vi "PH_SHS_Analysis.Draw Image.vi"(0 "i ref in":refnum<vi>, 2 "Cam Image":T1, 5 "error in (no error)":errorcluster) -> (14 "i ref out":refnum<vi>, 19 "error out":errorcluster)   [LabVIEW 2014, in "PH_SHS_Analysis.lvlib"]
doc: "This VI draws the image to the GUI. Depending on the sequencer state, it writes the images also to the attributes or calculates the pixel sum."
uses:
  PH_SHS_Analysis.lvlib
  <vilib>/vision/Image Controls.llb/IMAQ Image.ctl
  <vilib>/vision/NI_Vision_Development_Module.lvlib
  User/Eisenbarth/SHS_v4/SHS_Analysis/SHS_Analysis.lvlib
  User/Eisenbarth/SHS_v4/SHS_Common/SHS_Common.lvlib
  PH_Img_BaseClass/PH_Img_BaseClass.lvlib
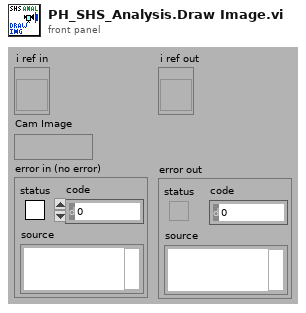
[diagram p1: front panel]
types:
  T1 = typedef "IMAQ Image.ctl" = refnum<image>
  T2 = typedef "Image Type" = u32
  T3 = typedef "PH_Img_BaseClass.lvlib/PH_Img_BaseClass.i attribute.ctl" = cluster{"GUI Refs":T4, "Timeout Image [ms]":i32, "Default Periodic Period [ms]":i32, "Camera":cluster{"Instancename":string, "Notifier":refnum<notifier>}, "Palette":T5, "Cam Settings":cluster{"Cam ID":string, "Gain":dbl, "Brightness":dbl, "Shutter":dbl, "Cam Info Failure":bool, "Mode":i32}}
  T4 = typedef "PH_Img_BaseClass.lvlib/PH_Img_BaseClass.GUI Refs.ctl" = cluster{"Timeout":refnum<vi>, "Image":refnum<vi>, "Palette":refnum<vi>, "Timeout Set":refnum<vi>}
  T5 = typedef "PH_Img_BaseClass.lvlib/PH_Img_BaseClass.Palette.ctl" = i32
  T6 = typedef "PH_SHS_Analysis.lvlib/PH_SHS_Analysis.i attribute.ctl" = cluster{"GUI Refs":cluster{"Delete":refnum<vi>, "Global On":refnum<vi>, "Cam Source":refnum<vi>, "Calibration Data File":refnum<vi>, "Calibration status":refnum<vi>, "Show overlay":refnum<vi>, "SHS Device Config":refnum<vi>, "Result":refnum<vi>, "Consider Tilt":refnum<vi>, "Working Reference":refnum<vi>, "Remove Tilt":refnum<vi>, "Take Cali  Reference":refnum<vi>, "Publishing Data Status":refnum<vi>, "Calibration Data":refnum<vi>}, "Calibration":cluster{"Status":T7, "Data":T8, "File":path}, "Result":T13, "Image":T1, "SHS Device Config":T16, "Show Overlay":bool, "GradientZernikeMatrix":dbl[][], "Consider Tilt":bool, "Working Reference":T9, "Zernicke Service ID":i32, "PSDB Image":T1}
  T7 = typedef "PH_StatusHandler.lvlib/PH_StatusHandler.Status.ctl" = i16
  T8 = typedef "PH_SHS_Analysis_Calibrator.lvlib/PH_SHS_Analysis_Calibrator.Analysis Calibration Data.ctl" = cluster{"Date":string, "Time":string, "Cam Settings":cluster{"Cam ID":string, "Gain":dbl, "Brightness":dbl, "Shutter":dbl, "Cam Error":bool, "Mode":i32}, "SHS Reference Result":T9, "Pixel Size":dbl, "MLA Pitch":dbl, "Method":enum16{"automatic", "manual"}, "Calibration Data calculated":bool, "No Problems at calculation?":bool, "error out":errorcluster}
  T9 = typedef "SHS_Common.lvlib/SHSReference.ctl" = cluster{"Reference":T10[][], "Lens Array Pitch [px]":dbl}
  T10 = typedef "SHS_Common.lvlib/ReferencePoint.ctl" = cluster{"Rect":T11, "Point":T12}
  T11 = typedef "SHS_Common.lvlib/Rectangle.ctl" = cluster{"Left":i32, "Top":i32, "Right":i32, "Bottom":i32}
  T12 = typedef "SHS_Common.lvlib/Point.ctl" = cluster{"x":dbl, "y":dbl, "valid?":bool, "weight":dbl}
  T13 = typedef "PH_SHS_Analysis.lvlib/PH_SHS_Analysis.Result.ctl" = cluster{"Time Stamp":timestamp, "Zernike Coefficients":T14, "PtV [lambda]":dbl, "Shifts":T15, "Measurement Quality":cluster{dbl, dbl, dbl}, "Measurement valid?":bool}
  T14 = typedef "PH_SHS_Analysis.lvlib/PH_SHS_Analysis.Zernike Coefficients.ctl" = cluster{"Tilt x":dbl, "Tilt y":dbl, "Defocus":dbl, "Astig 0°":dbl, "Astig 45°":dbl, "Coma x":dbl, "Coma y":dbl, "Spherical":dbl, "Trefoil 0°":dbl, "Trefoil 30°":dbl, "2nd Astig 0°":dbl, "2nd Astig 45°":dbl, "2nd Coma x":dbl, "2nd Coma y":dbl, "2nd Spherical":dbl}
  T15 = typedef "SHS_Common.lvlib/Shifts.ctl" = T12[][]
  T16 = typedef "SHS_Analysis.lvlib/SHS_DeviceConfig.ctl" = cluster{"focal length [m]":dbl, "pixel size [m/px]":dbl, "wavelength [m]":dbl}
  T17 = enum8{"Enabled", "Disabled", "Disabled and Grayed Out"}
  T18 = cluster{"Zernike Coeffcients[0]":dbl, "Zernike Coeffcients[1]":dbl, "Zernike Coeffcients[2]":dbl, "Zernike Coeffcients[3]":dbl, "Zernike Coeffcients[4]":dbl, "Zernike Coeffcients[5]":dbl, "Zernike Coeffcients[6]":dbl, "Zernike Coeffcients[7]":dbl, "Zernike Coeffcients[8]":dbl, "Zernike Coeffcients[9]":dbl, "Zernike Coeffcients[10]":dbl, "Zernike Coeffcients[11]":dbl, "Zernike Coeffcients[12]":dbl, "Zernike Coeffcients[13]":dbl, "Zernike Coeffcients[14]":dbl}
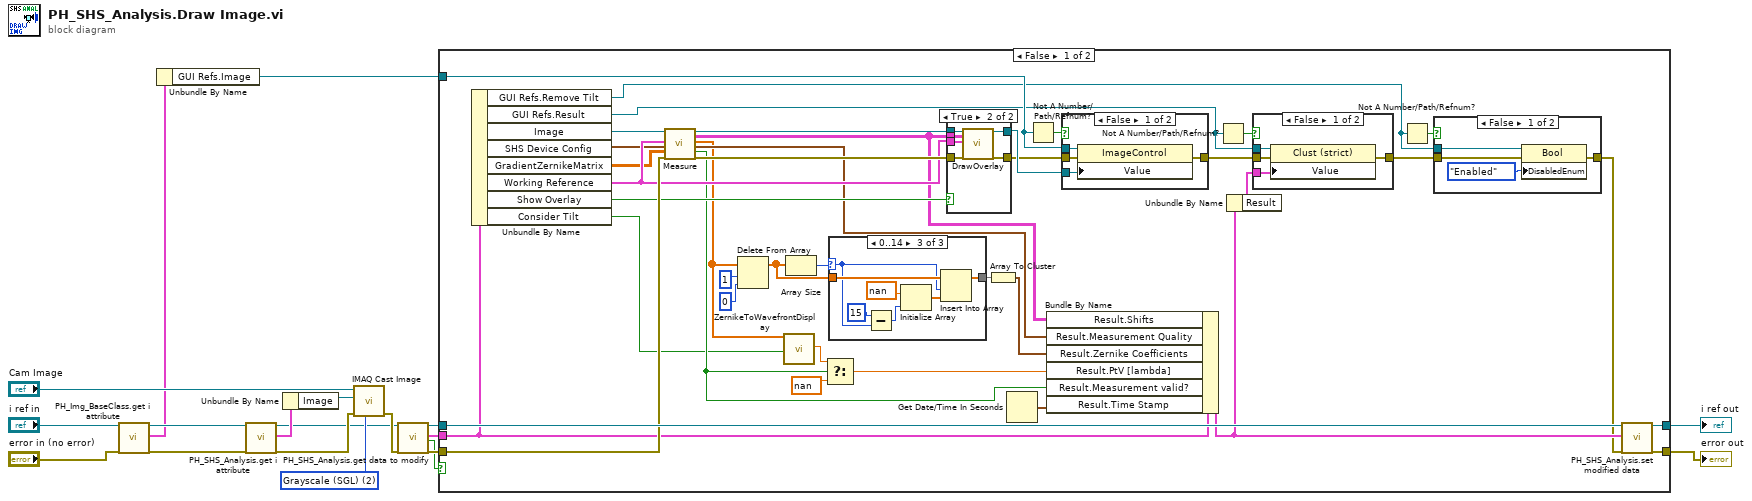
[diagram p0: block diagram]
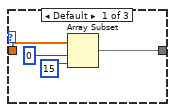
[diagram p2: hidden frame]
diagram:
  w14 = T2 2 items=["Grayscale (U8)", "Grayscale (I16)", "Grayscale (SGL)", "Complex (CSG)", "RGB (U32)", "HSL (U32)", "RGB (U64)"] ("Image Type")
  n1 = call "PH_Img_BaseClass.get i attribute.vi"("i ref in"="i ref in", "error in (no error)"="error in (no error)") -> ("i ref out"=w5:refnum<vi>, "i attribute"=w2:T3, "error out"=w3:errorcluster)  [unwired: 15 in]
  n2 = Unbundle By Name(w2) -> ("GUI Refs.Image"=w1:refnum<vi>)
  n3 = call "PH_SHS_Analysis.get i attribute.vi"("i ref in"=w5, "error in (no error)"=w3) -> ("i ref out"=w12:refnum<vi>, "i attribute"=w16:T6, "error out"=w15:errorcluster)  [unwired: 15 in]
  n4 = Unbundle By Name(w16) -> ("Image"=w8:T1)
  n5 = call "IMAQ Cast Image"("Image Type"=w14, "error in (no error)"=w15, "Image Dst"=w8, "Image Src"="Cam Image") -> ("error out"=w13:errorcluster)  [unwired: 6 in, 1 out]
  n6 = call "PH_SHS_Analysis.get data to modify.vi"("i ref in"=w12, "error in (no error)"=w13) -> ("i ref out"=w11:refnum<vi>, "i attribute"=w10:T6, "timed out"=w7:bool, "error out"=w9:errorcluster)  [unwired: 14 in]
  n7 = case shown="False" w7 {
    tunnel: w11 -> [w59 w96]
    tunnel: w10 -> [w46 _]
    tunnel: w9 -> [w57 w95]
    tunnel: [w48 w96] -> w19
    tunnel: [w47 w95] -> w17
    tunnel: w1 -> [w22 _]
    frame False {
      n8 = Unbundle By Name(w46) -> ("GUI Refs.Remove Tilt"=w21:refnum<vi>, "GUI Refs.Result"=w20:refnum<vi>, "Image"=w35:T1, "SHS Device Config"=w51:T16, "GradientZernikeMatrix"=w49:dbl[][], "Working Reference"=w52:T9, "Show Overlay"=w50:bool, "Consider Tilt"=w36:bool)
      n9 = call "Measure.vi"("SHS Image"=w35, "SHS Reference"=w52, "SHS Device Config (dummy values)"=w51, "GradientZernikeMatrix"=w49, "error in (no error)"=w57) -> ("SHS Image out"=w56:T1, "Shifts"=w30:T15, "Zernike Coeffcients"=w23:dbl[], "Measurement Quality"=w41:cluster{dbl, dbl, dbl}, "Measurement valid?"=w40:bool, "error out"=w54:errorcluster)  [unwired: 9 in]
      n10 = Delete From Array(array=w23, length=1, index=0) -> (array with subset deleted=w26:dbl[])  [unwired: 1 out]
      n11 = call "ZernikeToWavefrontDisplay.vi"("Zernike Coeffcients"=w23, "Consider Tilt (false)"=w36) -> ("PtV [lambda]"=w43:dbl)  [unwired: 15 in, 2 out]
      n12 = Array Size(array=w26) -> (size(s)=w29:i32)
      n13 = Select(t=w43, s=w40, f=nan) -> (s? t:f=w44:dbl)
      n14 = case shown="0..14" w29 {
        selector: w29 -> [_ _ w66]
        tunnel: [w62 w64 w70] -> w27
        tunnel: w26 -> [w63 w64 w71]
        frame Default {
          n15 = Array Subset(array=w63, index=0, length=15) -> (w62:dbl[])
        }
        frame 15 {
        }
        frame 0..14 {
          n16 = Subtract(x=15, y=w66) -> (x-y=w68:i32)
          n17 = Initialize Array(nan ("element"), w68) -> (w67:dbl[])
          n18 = Insert Into Array(array=w71, index=w66, new element=w67) -> (w70:dbl[])
        }
      }
      n19 = case shown="True" w50 {
        tunnel: [w82 w89] -> w55
        tunnel: [w83 w88] -> w53
        tunnel: w54 -> [w83 w87]
        tunnel: w56 -> [w82 w86]
        tunnel: w30 -> [_ w85]
        tunnel: w52 -> [_ w84]
        frame False {
        }
        frame True {
          n20 = call "DrawOverlay.vi"("Image"=w86, "Shifts"=w85, "SHS Reference"=w84, "error in (no error)"=w87) -> ("Image Out"=w89:T1, "error out"=w88:errorcluster)  [unwired: 14 in]
        }
      }
      n21 = Array To Cluster(array=w27) -> (cluster=w28:T18)
      n22 = Get Date/Time In Seconds() -> (seconds since 1Jan1904=w45:timestamp)
      n23 = Not A Number/Path/Refnum?(number/path/refnum=w22) -> (NaN/Path/Refnum?=w58:bool)
      n24 = Bundle By Name(cluster=w46, "Result.Shifts"=w30, "Result.Measurement Quality"=w41, "Result.Zernike Coefficients"=w28, "Result.PtV [lambda]"=w44, "Result.Measurement valid?"=w40, "Result.Time Stamp"=w45) -> (w32:T6)
      n25 = case shown="False" w58 {
        tunnel: w22 -> [w93 _]
        tunnel: [w92 w94] -> w39
        tunnel: w55 -> [w91 _]
        tunnel: w53 -> [w90 w94]
        frame False {
          n26 = property class="ImageControl"(reference=w93, error in=w90, "Value"=w91) -> (error out=w92:errorcluster)  [unwired: 1 out]
        }
        frame True {
        }
      }
      n27 = Not A Number/Path/Refnum?(number/path/refnum=w20) -> (NaN/Path/Refnum?=w38:bool)
      n28 = Unbundle By Name(w32) -> ("Result"=w37:T13)
      n29 = case shown="False" w38 {
        tunnel: w20 -> [w80 _]
        tunnel: [w79 w81] -> w33
        tunnel: w37 -> [w78 _]
        tunnel: w39 -> [w77 w81]
        frame False {
          n30 = property class="Clust (strict)"(reference=w80, error in=w77, "Value"=w78) -> (error out=w79:errorcluster)  [unwired: 1 out]
        }
        frame True {
        }
      }
      n31 = Not A Number/Path/Refnum?(number/path/refnum=w21) -> (NaN/Path/Refnum?=w34:bool)
      n32 = case shown="False" w34 {
        tunnel: w33 -> [w75 w76]
        tunnel: [w74 w76] -> w31
        tunnel: w21 -> [w73 _]
        frame False {
          n33 = property class="Bool"(reference=w73, error in=w75, "DisabledEnum"=T17."Enabled" ("Disabled")) -> (error out=w74:errorcluster)  [unwired: 1 out]
        }
        frame True {
        }
      }
      n34 = call "PH_SHS_Analysis.set modified data.vi"("i ref in"=w59, "i attribute"=w32, "error in (no error)"=w31) -> ("i ref out"=w48:refnum<vi>, "error out"=w47:errorcluster)  [unwired: 15 in]
    }
    frame True {
    }
  }
  "error out" <- w17
  "i ref out" <- w19
